vi "BRig_Host_dataRunState__entryDelete__delDataPlot__v3.vi"(7 "input_idx":i32[](array[numeric]), 8 "input_col_dataPlot":u16, 9 "input_row_dataPlot":u16, 10 "input_nTrial":u16, 11 "input_dataPlot":u16[][](array[numeric])) -> (0 "output_arrTrials":bool, 3 "output_dataPlot":u16[][](array[numeric]), 4 "output_arrTrials_length":i32, 5 "output_idx":i32[](array[numeric]), 6 "output_arrTrials":i32[](array[numeric]))   [LabVIEW 2014]
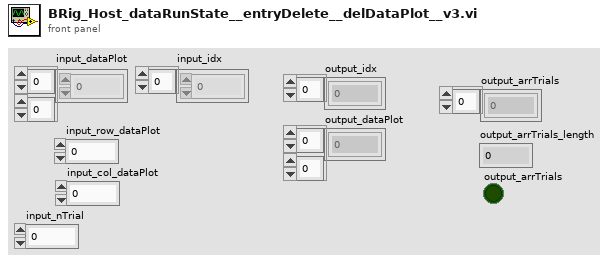
[diagram p1: front panel]
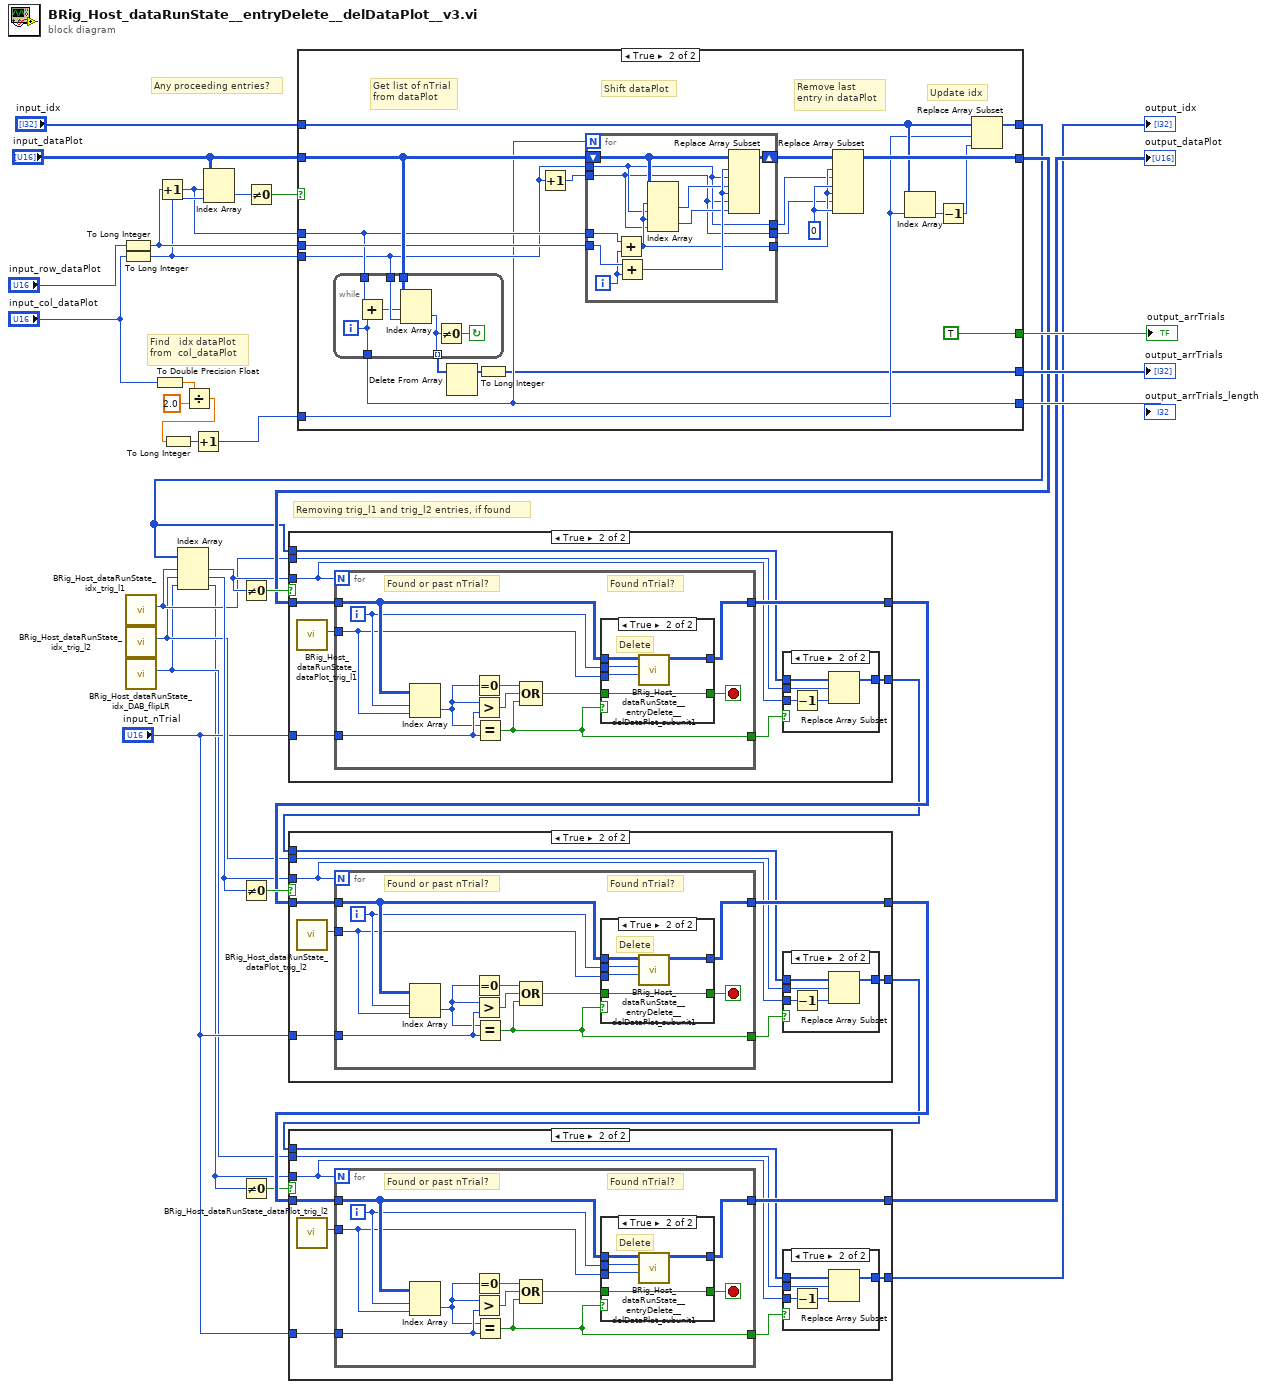
[diagram p0: block diagram]
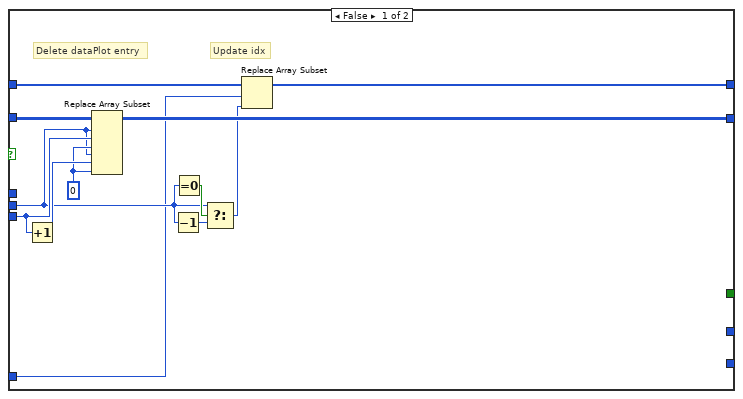
[diagram p11: hidden frame]
diagram:
  # "Removing trig_l1 and trig_l2 entries, if found"
  # "Find   idx dataPlot\nfrom  col_dataPlot"
  # "Any proceeding entries?"
  n1 = To Long Integer(number="input_row_dataPlot") -> (32bit integer=w31:i32)
  n2 = To Long Integer(number="input_col_dataPlot") -> (32bit integer=w30:i32)
  n3 = call "BRig_Host_dataRunState_idx_trig_l1.vi"() -> ("output_idx_trig_l1"=w10:i32)  [unwired: 11 in]
  n4 = call "BRig_Host_dataRunState_idx_trig_l2.vi"() -> ("output_idx_trig_l2"=w9:i32)  [unwired: 11 in]
  n5 = call "BRig_Host_dataRunState_idx_DAB_flipLR.vi"() -> ("output_idx_DAB_flipLR"=w2:i32)  [unwired: 11 in]
  n6 = To Double Precision Float(number="input_col_dataPlot") -> (double precision float=w28:dbl)
  n7 = Increment(x=w31) -> (x+1=w29:i32)
  n8 = Divide(x=w28, y=2.0) -> (x/y=w26:dbl)
  n9 = To Long Integer(number=w26) -> (32bit integer=w25:i32)
  n10 = Increment(x=w25) -> (x+1=w23:i32)
  n11 = Index Array(array="input_dataPlot", index (row)=w29, index (col)=w30) -> (element=w34:u16)
  n12 = Not Equal To 0?(x=w34) -> (x != 0?=w33:bool)
  n13 = case shown="True" w33 {
    tunnel: "input_dataPlot" -> [w47 w67]
    tunnel: "input_idx" -> [w42 w55]
    tunnel: w31 -> [w38 w66]
    tunnel: w30 -> [w43 w64]
    tunnel: [w44 w57] -> w18
    tunnel: [w41 w56] -> w15
    tunnel: w29 -> [_ w65]
    tunnel: w23 -> [w36 w52]
    tunnel: [_ w48] -> w22
    tunnel: [_ w51] -> w21
    tunnel: [_ TRUE] -> w20
    frame False {
      w45 = u16 0 ("new element/subarray")
      # "Update idx"
      # "Delete dataPlot entry"
      n14 = Increment(x=w43) -> (x+1=w46:i32)
      n15 = Replace Array Subset(array=w47, new element #1=w45, index (row) #1=w38, index (col) #1=w43, new element #2=w45, index (row) #2=w38, index (col) #2=w46) -> (w44:u16[][])
      n16 = Decrement(x=w38) -> (x-1=w39:i32)
      n17 = Equal To 0?(x=w38) -> (x = 0?=w40:bool)
      n18 = Select(t=w38, s=w40, f=w39) -> (s? t:f=w37:i32)
      n19 = Replace Array Subset(array=w42, new element=w37, index=w36) -> (w41:i32[])
    }
    frame True {
      w62 = u16 0 ("new element/subarray")
      # "Update idx"
      # "Remove last\nentry in dataPlot"
      # "Shift dataPlot"
      # "Get list of nTrial\nfrom dataPlot"
      n20 = while {
        tunnel: w67 -> [w86]
        tunnel: w65 -> [w83]
        tunnel: w64 -> [w85]
        tunnel: [w81] -> w68 mode=indexing
        tunnel: [w80] -> w51
        i -> [w80]
        stop <- w82 continue-if-true
        n21 = Add(x=w83, y=w80) -> (x+y=w84:i32)
        n22 = Index Array(array=w86, index (row)=w84, index (col)=w85) -> (element=w81:u16)
        n23 = Not Equal To 0?(x=w81) -> (x != 0?=w82:bool)
      }
      n24 = Delete From Array(array=w68) -> (array with subset deleted=w49:u16[])  [unwired: 2 in, 1 out]
      n25 = To Long Integer(number=w49) -> (32bit integer=w48:i32[])
      n26 = Increment(x=w64) -> (x+1=w63:i32)
      n27 = for {
        N: w51 -> [_]
        shift-right: [w79] -> w61
        shift-left: w67 -> [w78]
        tunnel: w66 -> [w77]
        tunnel: w65 -> [w75]
        tunnel: w64 -> [w70]
        tunnel: w63 -> [w69]
        tunnel: [w71] -> w60
        tunnel: [w70] -> w59
        tunnel: [w69] -> w58
        i -> [w76]
        n28 = Add(x=w75, y=w76) -> (x+y=w71:i32)
        n29 = Add(x=w77, y=w76) -> (x+y=w74:i32)
        n30 = Index Array(array=w78, index (row) #1=w71, index (col) #1=w70, index (row) #2=w71, index (col) #2=w69) -> (element #1=w73:u16, element #2=w72:u16)
        n31 = Replace Array Subset(array=w78, new element #1=w73, index (row) #1=w74, index (col) #1=w70, new element #2=w72, index (row) #2=w74, index (col) #2=w69) -> (w79:u16[][])
      }
      n32 = Replace Array Subset(array=w61, new element #1=w62, index (row) #1=w60, index (col) #1=w59, new element #2=w62, index (row) #2=w60, index (col) #2=w58) -> (w57:u16[][])
      n33 = Index Array(array=w55, index=w52) -> (element=w54:i32)
      n34 = Decrement(x=w54) -> (x-1=w53:i32)
      n35 = Replace Array Subset(array=w55, new element=w53, index=w52) -> (w56:i32[])
    }
  }
  "output_arrTrials" <- w22
  "output_arrTrials_length" <- w21
  "output_arrTrials" <- w20
  n36 = Index Array(array=w15, index #1=w10, index #2=w9, index #3=w2) -> (element #1=w16:i32, element #2=w12:i32, element #3=w1:i32)
  n37 = Not Equal To 0?(x=w16) -> (x != 0?=w19:bool)
  n38 = Not Equal To 0?(x=w12) -> (x != 0?=w14:bool)
  n39 = Not Equal To 0?(x=w1) -> (x != 0?=w3:bool)
  n40 = case shown="True" w19 {
    tunnel: w16 -> [_ w91]
    tunnel: w18 -> [w88 w97]
    tunnel: "input_nTrial" -> [_ w95]
    tunnel: [w88 w94] -> w13
    tunnel: w15 -> [w87 w92]
    tunnel: w10 -> [_ w90]
    tunnel: [w87 w89] -> w11
    frame False {
    }
    frame True {
      n41 = call "BRig_Host_dataRunState_dataPlot_trig_l1.vi"() -> ("output_idx_dataPlot_trig_l1"=w96:i32)  [unwired: 11 in]
      n42 = for {
        N: w91 -> [_]
        tunnel: w97 -> [w112]
        tunnel: w96 -> [w110]
        tunnel: w95 -> [w114]
        tunnel: [w108] -> w94
        tunnel: [w107] -> w93
        i -> [w111]
        stop <- w109 stop-if-true
        # "Found nTrial?"
        # "Found or past nTrial?"
        n43 = Index Array(array=w112, index (row)=w111, index (col)=w110) -> (element=w106:u16)
        n44 = Equal To 0?(x=w106) -> (x = 0?=w105:bool)
        n45 = Greater?(x=w106, y=w114) -> (0:w104:bool)
        n46 = Equal?(x=w106, y=w114) -> (x = y?=w107:bool)
        n47 = Compound Arithmetic op=OR(w105, w104, w107) -> (w113:bool)
        n48 = case shown="True" w107 {
          tunnel: w112 -> [w116 w121]
          tunnel: w111 -> [_ w120]
          tunnel: w110 -> [_ w119]
          tunnel: [w116 w118] -> w108
          tunnel: w113 -> [w115 w117]
          tunnel: [w115 w117] -> w109
          frame False {
          }
          frame True {
            # "Delete"
            n49 = call "BRig_Host_dataRunState__entryDelete__delDataPlot_subunit1.vi"("input_col_dataPlot"=w119, "input_row_dataPlot"=w120, "input_dataPlot"=w121) -> ("output_dataPlot"=w118:u16[][])  [unwired: 8 in]
          }
        }
      }
      n50 = case shown="True" w93 {
        tunnel: w92 -> [w98 w102]
        tunnel: w91 -> [_ w103]
        tunnel: w90 -> [_ w101]
        tunnel: [w98 w99] -> w89
        frame False {
        }
        frame True {
          n51 = Decrement(x=w103) -> (x-1=w100:i32)
          n52 = Replace Array Subset(array=w102, new element=w100, index=w101) -> (w99:i32[])
        }
      }
    }
  }
  n53 = case shown="True" w14 {
    tunnel: w12 -> [_ w127]
    tunnel: w13 -> [w123 w132]
    tunnel: "input_nTrial" -> [_ w131]
    tunnel: [w123 w130] -> w7
    tunnel: w11 -> [w122 w128]
    tunnel: w9 -> [_ w126]
    tunnel: [w122 w125] -> w6
    frame False {
    }
    frame True {
      n54 = call "BRig_Host_dataRunState_dataPlot_trig_l2.vi"() -> ("output_idx_dataPlot_trig_l2"=w124:i32)  [unwired: 11 in]
      n55 = for {
        N: w127 -> [_]
        tunnel: w132 -> [w147]
        tunnel: w124 -> [w145]
        tunnel: w131 -> [w149]
        tunnel: [w143] -> w130
        tunnel: [w142] -> w129
        i -> [w146]
        stop <- w144 stop-if-true
        # "Found nTrial?"
        # "Found or past nTrial?"
        n56 = Index Array(array=w147, index (row)=w146, index (col)=w145) -> (element=w141:u16)
        n57 = Equal To 0?(x=w141) -> (x = 0?=w140:bool)
        n58 = Greater?(x=w141, y=w149) -> (0:w139:bool)
        n59 = Equal?(x=w141, y=w149) -> (x = y?=w142:bool)
        n60 = Compound Arithmetic op=OR(w140, w139, w142) -> (w148:bool)
        n61 = case shown="True" w142 {
          tunnel: w147 -> [w151 w156]
          tunnel: w146 -> [_ w155]
          tunnel: w145 -> [_ w154]
          tunnel: [w151 w153] -> w143
          tunnel: w148 -> [w150 w152]
          tunnel: [w150 w152] -> w144
          frame False {
          }
          frame True {
            # "Delete"
            n62 = call "BRig_Host_dataRunState__entryDelete__delDataPlot_subunit1.vi"("input_col_dataPlot"=w154, "input_row_dataPlot"=w155, "input_dataPlot"=w156) -> ("output_dataPlot"=w153:u16[][])  [unwired: 8 in]
          }
        }
      }
      n63 = case shown="True" w129 {
        tunnel: w128 -> [w133 w137]
        tunnel: w127 -> [_ w138]
        tunnel: w126 -> [_ w136]
        tunnel: [w133 w134] -> w125
        frame False {
        }
        frame True {
          n64 = Decrement(x=w138) -> (x-1=w135:i32)
          n65 = Replace Array Subset(array=w137, new element=w135, index=w136) -> (w134:i32[])
        }
      }
    }
  }
  n66 = case shown="True" w3 {
    tunnel: w1 -> [_ w162]
    tunnel: w7 -> [w158 w167]
    tunnel: "input_nTrial" -> [_ w166]
    tunnel: [w158 w165] -> w8
    tunnel: w6 -> [w157 w163]
    tunnel: w2 -> [_ w161]
    tunnel: [w157 w160] -> w4
    frame False {
    }
    frame True {
      n67 = call "BRig_Host_dataRunState_dataPlot_trig_l2.vi"() -> ("output_idx_dataPlot_trig_l2"=w159:i32)  [unwired: 11 in]
      n68 = for {
        N: w162 -> [_]
        tunnel: w167 -> [w182]
        tunnel: w159 -> [w180]
        tunnel: w166 -> [w184]
        tunnel: [w178] -> w165
        tunnel: [w177] -> w164
        i -> [w181]
        stop <- w179 stop-if-true
        # "Found nTrial?"
        # "Found or past nTrial?"
        n69 = Index Array(array=w182, index (row)=w181, index (col)=w180) -> (element=w176:u16)
        n70 = Equal To 0?(x=w176) -> (x = 0?=w175:bool)
        n71 = Greater?(x=w176, y=w184) -> (0:w174:bool)
        n72 = Equal?(x=w176, y=w184) -> (x = y?=w177:bool)
        n73 = Compound Arithmetic op=OR(w175, w174, w177) -> (w183:bool)
        n74 = case shown="True" w177 {
          tunnel: w182 -> [w186 w191]
          tunnel: w181 -> [_ w190]
          tunnel: w180 -> [_ w189]
          tunnel: [w186 w188] -> w178
          tunnel: w183 -> [w185 w187]
          tunnel: [w185 w187] -> w179
          frame False {
          }
          frame True {
            # "Delete"
            n75 = call "BRig_Host_dataRunState__entryDelete__delDataPlot_subunit1.vi"("input_col_dataPlot"=w189, "input_row_dataPlot"=w190, "input_dataPlot"=w191) -> ("output_dataPlot"=w188:u16[][])  [unwired: 8 in]
          }
        }
      }
      n76 = case shown="True" w164 {
        tunnel: w163 -> [w168 w172]
        tunnel: w162 -> [_ w173]
        tunnel: w161 -> [_ w171]
        tunnel: [w168 w169] -> w160
        frame False {
        }
        frame True {
          n77 = Decrement(x=w173) -> (x-1=w170:i32)
          n78 = Replace Array Subset(array=w172, new element=w170, index=w171) -> (w169:i32[])
        }
      }
    }
  }
  "output_idx" <- w4
  "output_dataPlot" <- w8
